vi "TagDB-Change Detector.vi"   [LabVIEW 2017, in "TagDB.lvlib"]
uses:
  TagDB.lvlib
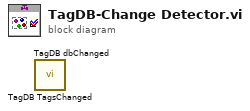
[diagram p0: block diagram]
diagram:
  n1 = call "TagDB TagsChanged.vi"() -> ()  [unwired: 9 in, 3 out]
  n2 = call "TagDB dbChanged.vi"() -> ()  [unwired: 9 in, 3 out]
